vi "Sharp Read (SubVI).vi"(7 "error in (no error)":errorcluster) -> (18 "BL (B/AI2 (Pin 7))":dbl, 19 "LB (B/AI3 (Pin 9))":dbl, 21 "LF (A/AI0 (Pin 3))":dbl, 22 "FL (A/AI1 (Pin 5))":dbl, 23 "FR (A/AI2 (Pin 7))":dbl, 24 "RF (C/AI0 (AI0))":dbl, 25 "RB (B/AI0 (Pin 3))":dbl, 26 "BR (B/AI1 (Pin 5))":dbl, 27 "error out":errorcluster)   [LabVIEW 2017]
doc: "Reads values from one or more analog input channels.\n--------------------\n\nThis Express VI is configured as follows:\n\nNode name: Analog input (1 sample)\nChannel: A/AI0 (Pin 3) ; Custom Name: LF\nChannel: A/AI1 (Pin 5) ; Custom Name: FL\nChannel: A/AI2 (Pin 7) ; Custom Name: FR\nChannel: C/AI0 (AI0) ; Custom Name: RF\nChannel: B/AI0 (Pin 3) ; Custom Name: RB\nChannel: B/AI1 (Pin 5) ; Custom Name: BR\nChannel: B/AI2 (Pin 7) ; Custom Name: BL\nChannel: B/AI3 (Pin 9) ; Custom Name: LB"
uses:
  <vilib>/myRIO/Common/Instrument Driver Framework/myRIO v1.0/AI/vis/myRIO v1.0 Read AI.vi
  <vilib>/Utility/error.llb/Error Cluster From Error Code.vi
  <vilib>/myRIO/Instrument Drivers/Onboard IO/AI/AI.lvlib
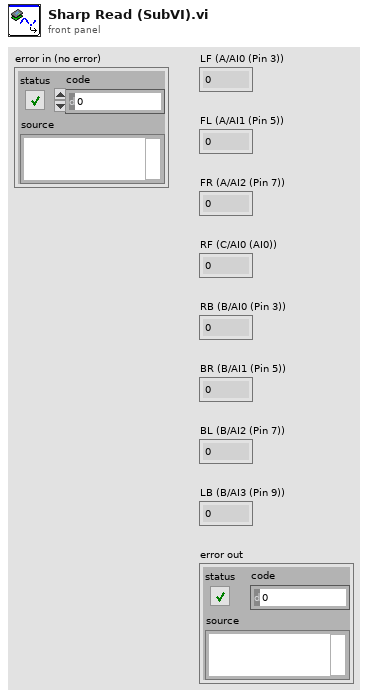
[diagram p1: front panel]
types:
  T1 = typedef "AI.lvlib/AI Reference.ctl" = cluster{"myRIO Reference":T2, "AI Channels List":T6, "AI Scaling Constants List":T8}
  T2 = typedef "myRIO Generic Hardware Reference.ctl" = cluster{"myRIO Model":T3, "myRIO Hardware Reference":T4}
  T3 = typedef "Hardware Version Enum.ctl" = enum16{"Unknown", "myRIO-1900", "myRIO-1950", "roboRIO", "NI ELVIS RIO CM"}
  T4 = typedef "myRIO v1.0 Reference.ctl" = cluster{"Generic FPGA Reference":T5, "Allow multiple opens":bool}
  T5 = typedef "Generic FPGA Reference.ctl" = refnum<k20>
  T6 = typedef "AI Channels List.ctl" = T7[]
  T7 = typedef "AI Channels Enum.ctl" = enum16{"Not Connected", "AudioIn/Left", "AudioIn/Right", "C/AI0", "C/AI1", "A/AI0", "A/AI1", "A/AI2", "A/AI3", "B/AI0", "B/AI1", "B/AI2", "B/AI3", "AI/AI0", "AI/AI1", "AI/AI2", "AI/AI3"}
  T8 = typedef "Analog Scaling Constants List.ctl" = T9[]
  T9 = typedef "Analog Scaling Constants.ctl" = cluster{"LSB Weight (Volts)":dbl, "Offset (Volts)":dbl, "Signed?":bool}
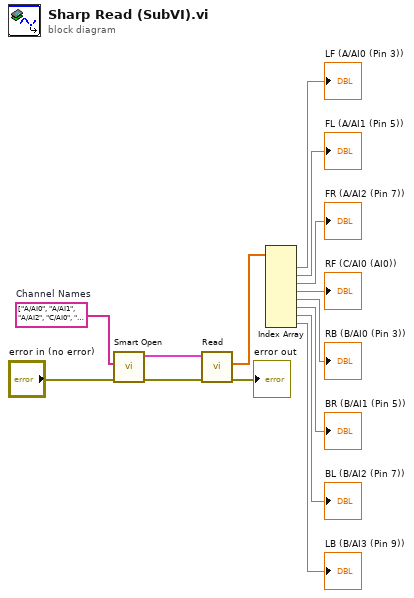
[diagram p0: block diagram]
diagram:
  w14 = tag[] ["A/AI0", "A/AI1", "A/AI2", "C/AI0", "B/AI0", "B/AI1", "B/AI2", "B/AI3"]  # Channel Names
  n1 = call <vilib>:"Smart Open.vi"("error in (no error)"="error in (no error)", "Channel Names"=w14) -> ("error out"=w2:errorcluster, "AI Ref Out"=w3:T1)  [unwired: 8 in]
  n2 = call <vilib>:"Read.vi"("error in (no error)"=w2, "AI Ref In"=w3) -> ("error out"=→"error out":errorcluster, "Values"=w13:dbl[])  [unwired: 7 in, 1 out]
  n3 = Index Array(array=w13) -> (element #1=→"LF (A/AI0 (Pin 3))":dbl, element #2=→"FL (A/AI1 (Pin 5))":dbl, element #3=→"FR (A/AI2 (Pin 7))":dbl, element #4=→"RF (C/AI0 (AI0))":dbl, element #5=→"RB (B/AI0 (Pin 3))":dbl, element #6=→"BR (B/AI1 (Pin 5))":dbl, element #7=→"BL (B/AI2 (Pin 7))":dbl, element #8=→"LB (B/AI3 (Pin 9))":dbl)  [unwired: 8 in]
